vi "09 LV - Workbook from template.vi"() -> ()   [LabVIEW 2020]
uses:
  client/client.lvlib
  client/Client/Client.lvclass
  client/List/List.lvclass
  client/Workbook/Workbook.lvclass
panel:
  out "workbook names":string[](array[string])
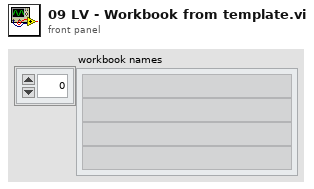
[diagram p1: front panel]
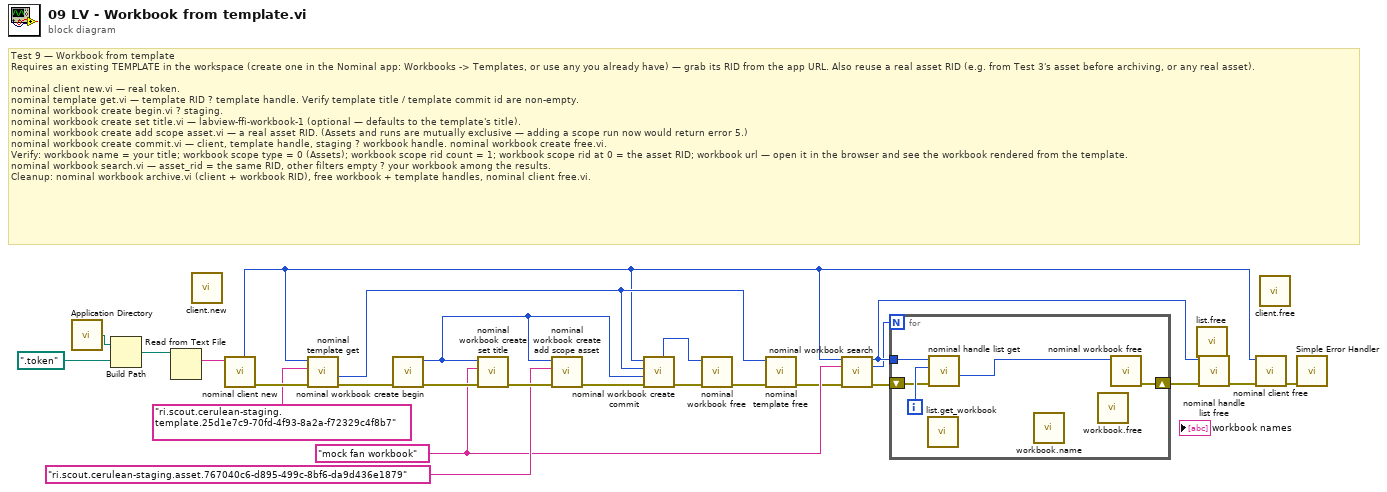
[diagram p0: block diagram]
diagram:
  w8 = "mock fan workbook" ("title")
  # "Test 9 — Workbook from template\nRequires an existing TEMPLATE in the workspace (create one in the Nominal app: Workbooks -> Templates, or use any you already have) — grab its RID from the app URL. Also reuse a real asset RID (e.g. from Test 3's asset before archiving, or any real asset).\n\nnominal client new.vi — real token.\nnominal template get.vi — template RID ? template handle. Verify template title / template commit id are non-empty.\nnominal workbook create begin.vi ? staging.\nnominal workbook create set title.vi — labview-ffi-workbook-1 (optional — defaults to the template's title).\nnominal workbook create add scope asset.vi — a real asset RID. (Assets and runs are mutually exclusive — adding a scope run now would return error 5.)\nnominal workbook create commit.vi — client, template handle, staging ? workbook handle. nominal workbook create free.vi.\nVerify: workbook name = your title; workbook scope type = 0 (Assets); workbook scope rid count = 1; workbook scope rid at 0 = the asset RID; workbook url — open it in the browser and see the workbook rendered from the template.\nnominal workbook search.vi — asset_rid = the same RID, other filters empty ? your workbook among the results.\nCleanup: nominal workbook archive.vi (client + workbook RID), free workbook + template handles, nominal client free.vi."
  n1 = call <vilib>:"Application Directory.vi"() -> ("Application Directory"=w25:path)
  n2 = Build Path(base path=w25, name or relative path=path ".token") -> (appended path=w23:path)
  n3 = Read from Text File(file (use dialog)=w23) -> (text=w22:string)  [unwired: 3 in, 3 out]
  n4 = call "client.new.vi"() -> ()  [unwired: 10 in, 2 out]
  n5 = call "nominal client new.vi"("token"=w22) -> ("error out"=w20:errorcluster, "out_client out"=w7:i32)  [unwired: 8 in, 1 out]
  n6 = call "nominal template get.vi"("error in (no error)"=w20, "rid"="ri.scout.cerulean-staging.template.25d1e7c9-70fd-4f93-8a2a-f72329c4f8b7", "client"=w7) -> ("error out"=w19:errorcluster, "out_template out"=w14:i32)  [unwired: 6 in, 1 out]
  n7 = call "nominal workbook create begin.vi"("error in (no error)"=w19) -> ("error out"=w18:errorcluster, "out_staging out"=w15:i32)  [unwired: 8 in, 1 out]
  n8 = call "nominal workbook create set title.vi"("error in (no error)"=w18, "title"=w8, "staging"=w15) -> ("error out"=w17:errorcluster)  [unwired: 7 in, 1 out]
  n9 = call "nominal workbook create add scope asset.vi"("error in (no error)"=w17, "asset_rid"="ri.scout.cerulean-staging.asset.767040c6-d895-499c-8bf6-da9d436e1879" ("title"), "staging"=w15) -> ("error out"=w16:errorcluster)  [unwired: 7 in, 1 out]
  n10 = call "nominal workbook create commit.vi"("error in (no error)"=w16, "staging"=w15, "template_"=w14, "client"=w7) -> ("error out"=w11:errorcluster, "out_workbook out"=w13:i32)  [unwired: 5 in, 1 out]
  n11 = call "nominal workbook free.vi"("error in (no error)"=w11, "workbook"=w13) -> ("error out"=w12:errorcluster)  [unwired: 8 in, 1 out]
  n12 = call "nominal template free.vi"("error in (no error)"=w12, "template_"=w14) -> ("error out"=w6:errorcluster)  [unwired: 8 in, 1 out]
  n13 = call "nominal workbook search.vi"("client"=w7, "search_text"=w8, "error in (no error)"=w6) -> ("out_list out"=w4:i32, "out_count out"=w1:u32, "error out"=w5:errorcluster)  [unwired: 9 in, 1 out]
  n14 = for {
    N: w1 -> [_]
    tunnel: w4 -> [w30]
    shift-right: [w27] -> w3
    shift-left: w5 -> [w28]
    i -> [w29]
    n15 = call "list.get_workbook.vi"() -> ()  [unwired: 9 in, 3 out]
    n16 = call "nominal handle list get.vi"("error in (no error)"=w28, "index"=w29, "list"=w30) -> ("out_handle out"=w26:i32)  [unwired: 6 in, 2 out]
    n17 = call "workbook.name.vi"() -> ()  [unwired: 9 in, 3 out]
    n18 = call "workbook.free.vi"() -> ()  [unwired: 11 in, 1 out]
    n19 = call "nominal workbook free.vi"("workbook"=w26) -> ("error out"=w27:errorcluster)  [unwired: 9 in, 1 out]
  }
  n20 = call "list.free.vi"() -> ()  [unwired: 11 in, 1 out]
  n21 = call "nominal handle list free.vi"("error in (no error)"=w3, "list"=w4) -> ("error out"=w2:errorcluster)  [unwired: 8 in, 1 out]
  n22 = call "nominal client free.vi"("error in (no error)"=w2, "client"=w7) -> ("error out"=w21:errorcluster)  [unwired: 8 in, 1 out]
  n23 = call "client.free.vi"() -> ()  [unwired: 11 in, 1 out]
  n24 = call <vilib>:"Simple Error Handler.vi"("error in (no error)"=w21) -> ()  [unwired: 4 in, 5 out]
